vi "Agilent PWM Initialize.vi"(8 "error in (no error)":errorcluster, 11 "Configuration":T2={"BusType"=enum."GPIB", "GPIB Bus"=0, "GPIB Address"=16, "IP"=0, "COM"=1, "Baud Rate"=enum."9600", "USB Device"=0, "Instrument S\\N"="", "SCIL Address"=16} {"USB Device" max=31 step=1}) -> (0 "error out":errorcluster {"code" format="%.0x"}, 3 "VISA Resource Name":refnum<visa-resource-name>, 5 "Agilent PWM":T1)   [LabVIEW 2011]
uses:
  PWM Configuration.ctl
  TypeDefs/Agilent PWM Instrument Info.ctl
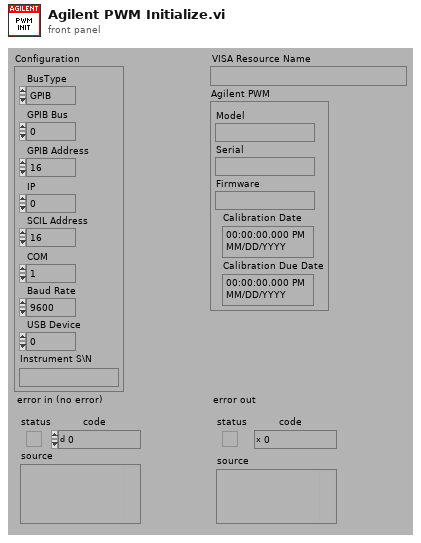
[diagram p1: front panel]
types:
  T1 = typedef "Agilent PWM Instrument Info.ctl" = cluster{"Model":string, "Serial":string, "Firmware":string, "Calibration Date":timestamp, "Calibration Due Date":timestamp}
  T2 = typedef "PWM Configuration.ctl" = cluster{"BusType":enum32{"GPIB", "LAN/IP", "Serial", "USB"}, "GPIB Bus":i32, "GPIB Address":i32, "IP":u32, "COM":i32, "Baud Rate":enum32{"300", "600", "1200", "2400", "4800", "9600"}, "USB Device":u32, "Instrument S\\N":string, "SCIL Address":i32}
  T3 = enum32{"300", "600", "1200", "2400", "4800", "9600"}
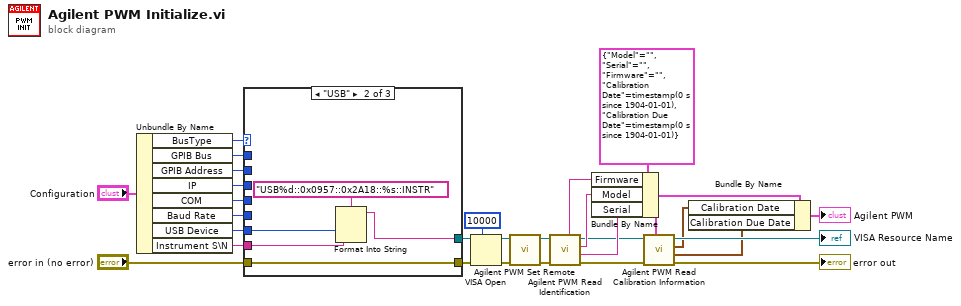
[diagram p0: block diagram]
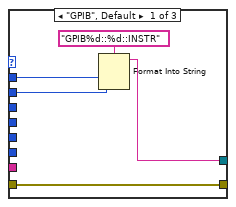
[diagram p2: hidden frame]
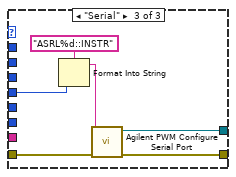
[diagram p3: hidden frame]
diagram:
  n1 = Unbundle By Name("Configuration") -> ("BusType"=w28:enum32{"GPIB", "LAN/IP", "Serial", "USB"}, "GPIB Bus"=w27:i32, "GPIB Address"=w26:i32, "IP"=w25:u32, "COM"=w24:i32, "Baud Rate"=w22:T3, "USB Device"=w10:u32, "Instrument S\\N"=w9:string)
  n2 = case shown="\"USB\"" w28 {
    tunnel: "error in (no error)" -> [w31 w38 w42]
    tunnel: w27 -> [w34 _ _]
    tunnel: w26 -> [w33 _ _]
    tunnel: w25 -> [_ _ _]
    tunnel: w24 -> [_ _ w44]
    tunnel: w22 -> [_ _ _]
    tunnel: [w31 w38 w41] -> w16
    tunnel: [w30 w37 w43] -> w15
    tunnel: w10 -> [_ w36 _]
    tunnel: w9 -> [_ w35 _]
    frame "GPIB", Default {
      n3 = Format Into String(format string="GPIB%d::%d::INSTR", w34, w33) -> (resulting string=w30:string)  [unwired: 2 in, 1 out]
    }
    frame "USB" {
      n4 = Format Into String(format string="USB%d::0x0957::0x2A18::%s::INSTR", w36, w35) -> (resulting string=w37:string)  [unwired: 2 in, 1 out]
    }
    frame "Serial" {
      n5 = Format Into String(format string="ASRL%d::INSTR", w44) -> (resulting string=w40:string)  [unwired: 2 in, 1 out]
      n6 = call "Agilent PWM Configure Serial Port.vi"("error in (no error)"=w42, "VISA Resource Name"=w40) -> ("error out"=w41:errorcluster, "dup VISA Resource Name"=w43:refnum<visa-resource-name>)  [unwired: 8 out]
    }
  }
  n7 = VISA Open(timeout (0)=u32 10000 ("VISA Open timeout (0)"), error in (no error)=w16, VISA resource name=w15) -> (VISA resource name=w11:refnum<visa-resource-name>, error out=w12:errorcluster)  [unwired: 2 out]
  n8 = call "Agilent PWM Set Remote.vi"("error in (no error)"=w12, "VISA Resource Name"=w11) -> ("error out"=w14:errorcluster, "dup VISA Resource Name"=w13:refnum<visa-resource-name>)  [unwired: 8 out]
  n9 = call "Agilent PWM Read Identification.vi"("error in (no error)"=w14, "VISA Resource Name"=w13) -> ("error out"=w8:errorcluster, "Serial Number"=w20:string, "Model"=w19:string, "dup VISA Resource Name"=w7:refnum<visa-resource-name>, "Firmware"=w21:string)  [unwired: 5 out]
  n10 = Bundle By Name(cluster=T1 {"Model"="", "Serial"="", "Firmware"="", "Calibration Date"=timestamp(0 s since 1904-01-01), "Calibration Due Date"=timestamp(0 s since 1904-01-01)} ("Agilent VNA"), "Firmware"=w21, "Model"=w19, "Serial"=w20) -> (w4:T1)
  n11 = call "Agilent PWM Read Calibration Information.vi"("Agilent PWM"=w4, "error in (no error)"=w8, "VISA Resource Name"=w7) -> ("error out"=→"error out":errorcluster, "Calibration Due Date"=w1:timestamp, "Calibration Date"=w2:timestamp, "dup VISA Resource Name"=→"VISA Resource Name":refnum<visa-resource-name>)  [unwired: 5 in]
  n12 = Bundle By Name(cluster=w4, "Calibration Date"=w2, "Calibration Due Date"=w1) -> (→"Agilent PWM":T1)
